vi "Channel_Start Wfms.vi"(8 "error in (no error)":errorcluster, 11 "Channel in":refnum<class "Channel.lvclass">) -> (0 "error out":errorcluster, 3 "Channel out":refnum<class "Channel.lvclass">)   [LabVIEW 2023, in "Channel.lvclass"]
doc: "Based on the waveform references given, start and open a waveform session with the reference."
uses:
  Channel.lvclass
  Channel.lvclass/Channel.ctl
  <vilib>/NI VeriStand/Custom Device Waveform API/Single Waveform Read (DBL)/NI VeriStand - Open Single Waveform Read Session (DBL).vi
  <vilib>/NI VeriStand/Custom Device Waveform API/Single Waveform Read (DBL)/Single Waveform Read (DBL).lvclass
  <vilib>/NI VeriStand/Custom Device Waveform API/NI_VS Custom Device Waveform API.lvlib
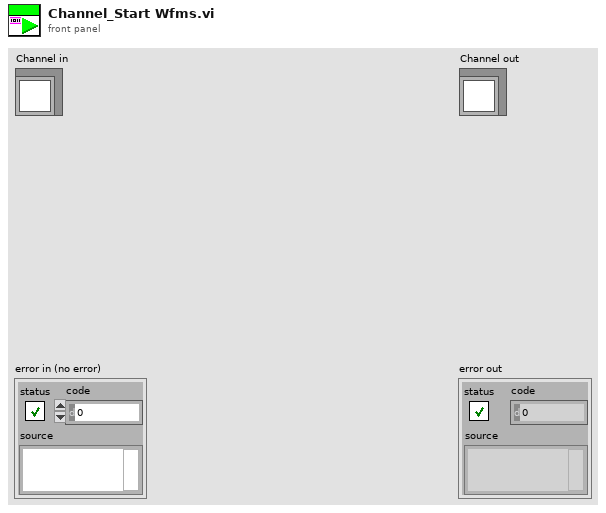
[diagram p1: front panel]
types:
  T1 = typedef "Custom Device API.lvlib/Data Reference.ctl" = i32
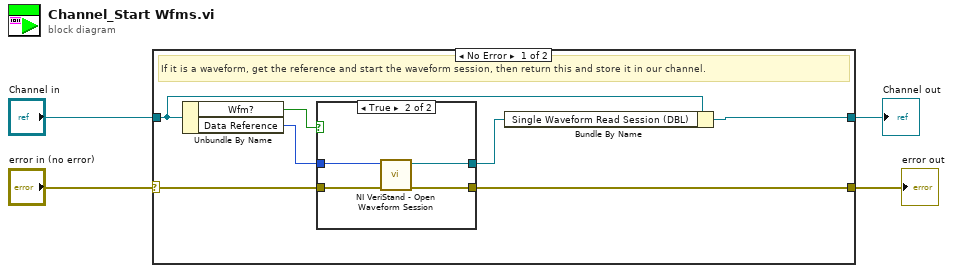
[diagram p0: block diagram]
diagram:
  n1 = case shown="No Error" "error in (no error)" {
    selector: "error in (no error)" -> [w10 w18]
    tunnel: [w9 w18] -> w3
    tunnel: [w7 w17] -> w1
    tunnel: "Channel in" -> [w8 w17]
    frame No Error {
      # "If it is a waveform, get the reference and start the waveform session, then return this and store it in our channel."
      n2 = Unbundle By Name(w8) -> ("Wfm?"=w6:bool, "Data Reference"=w11:T1)
      n3 = case shown="True" w6 {
        tunnel: w11 -> [_ w16]
        tunnel: w10 -> [w12 w15]
        tunnel: [w12 w14] -> w9
        tunnel: [_ w13] -> w5
        frame False {
        }
        frame True {
          n4 = call-poly <vilib>:"NI VeriStand - Open Waveform Session.vi"("error in (no error)"=w15, "DBL Waveform Data Reference"=w16) -> ("error out"=w14:errorcluster, "Single Waveform Read Session (DBL)"=w13:refnum<class "Single Waveform Read (DBL).lvclass">)  [unwired: 8 in]
        }
      }
      n5 = Bundle By Name(cluster=w8, "Single Waveform Read Session (DBL)"=w5) -> (w7:refnum<class "Channel.lvclass">)
    }
    frame Error {
    }
  }
  "error out" <- w3
  "Channel out" <- w1
